vi "ErrorCheckHWI.vi"(8 "error in (no error)":errorcluster, 11 "Agilent ESG in":refnum<class "Agilent ESG.lvclass">) -> (0 "error out":errorcluster, 3 "Agilent ESG out":refnum<class "Agilent ESG.lvclass">)   [LabVIEW 2013, in "Agilent ESG.lvclass"]
uses:
  Agilent ESG.lvclass
  Device/Device.lvclass
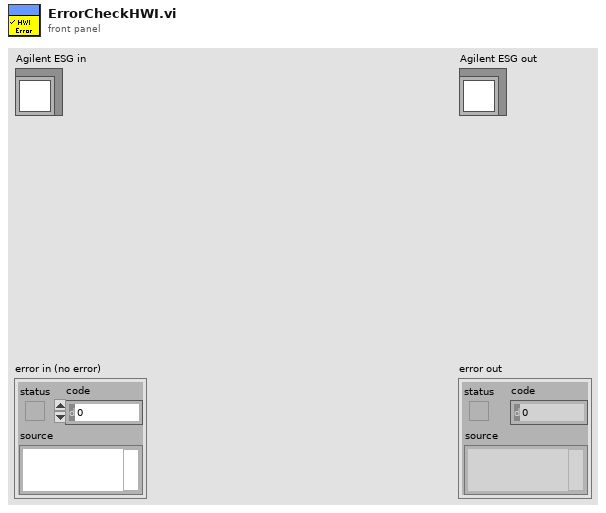
[diagram p1: front panel]
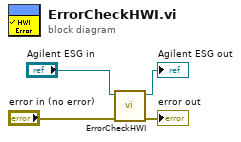
[diagram p0: block diagram]
diagram:
  n1 = call-parent "ErrorCheckHWI.vi"("error in (no error)"="error in (no error)", "Device in"="Agilent ESG in") -> ("error out"=→"error out":errorcluster, "Device out"=→"Agilent ESG out":refnum<class "Agilent ESG.lvclass">)  [unwired: 8 in]
